vi "niLvFpga_StartFifo_sbRIO-9603.vi"(0 "session in":u32, 5 "channel":u32, 11 "error in":errorcluster) -> (4 "session out":u32, 15 "error out":errorcluster)   [LabVIEW 2020]
uses:
  <vilib>/rvi/interface/common/niFpgaWaitOnOcc.vi
  NiFpgaLv.dll
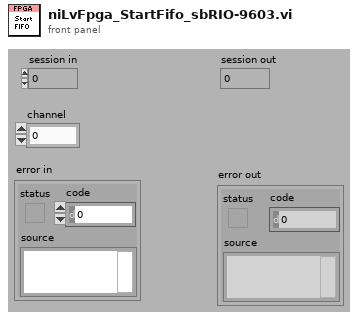
[diagram p1: front panel]
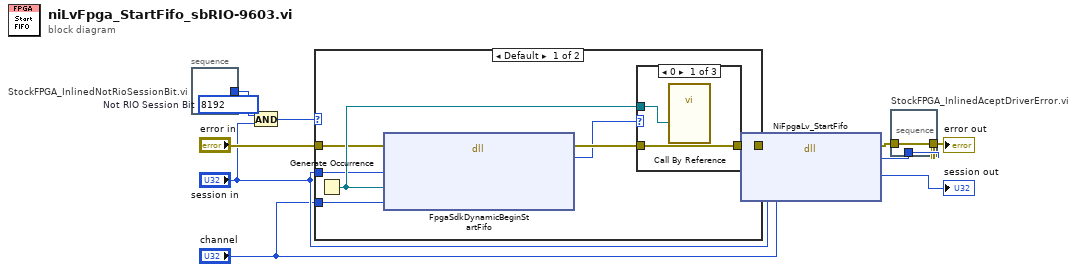
[diagram p0: block diagram]
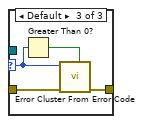
[diagram p4: hidden frame]
diagram:
  n1 = stacked-sequence "StockFPGA_InlinedNotRioSessionBit.vi" {
    tunnel: [w11] -> w3
    frame #0 {
      w11 = u32 8192  # Not RIO Session Bit
    }
  }
  n2 = And(x=w3, y="session in") -> (x .and. y?=w6:u32)
  n3 = case shown="Default" w6 {
    tunnel: "error in" -> [w15 w26]
    tunnel: [w14 w26] -> w4
    tunnel: "session in" -> [w13 _]
    tunnel: "channel" -> [w12 _]
    frame Default {
      n4 = Generate Occurrence() -> (w18:refnum<k4>)
      n5 = dll-call lib="LabVIEW" fn="FpgaSdkDynamicBeginStartFifo"(error in=w15, "session"=w13, "occurrence"=w18, "channel"=w12) -> (error out=w17:errorcluster, "status"=w16:i32)  [unwired: 5 in, 1 out]
      n6 = case shown="0" w16 {
        selector: w16 -> [_ _ w22]
        tunnel: [w20 w21 w24] -> w14
        tunnel: w17 -> [w20 w21 w25]
        tunnel: w18 -> [w19 _ _]
        frame 0 {
          n7 = call-by-ref "?"("occurrence"=w19) -> ()  [unwired: 16 in, 3 out]
        }
        frame -61167 {
          # "emulation case intentionally ignoring error"
        }
        frame Default {
          n8 = Greater Than 0?(x=w22) -> (x > 0?=w23:bool)
          n9 = call <vilib>:"Error Cluster From Error Code.vi"("is warning? (False)"=w23, "error in (no error)"=w25, "error code (0)"=w22) -> ("error out"=w24:errorcluster)  [unwired: 6 in]
        }
      }
    }
    frame 0 {
    }
  }
  n10 = dll-call lib="NiFpgaLv.*" fn="NiFpgaLv_StartFifo" label="niLvFpgaStartFifo"(error in=w4, "sessionID"="session in", "channel"="channel") -> (error out=w9:errorcluster, "status"=w7:i32, "sessionID"=→"session out":u32)  [unwired: 3 in, 1 out]
  n11 = stacked-sequence "StockFPGA_InlinedAceptDriverError.vi" {
    tunnel: w9 -> [w27]
    tunnel: w7 -> [w29]
    tunnel: [w28] -> w8
    frame #0 {
      n12 = case shown="Default" w29 {
        selector: w29 -> [_ w31]
        tunnel: [w30 w33] -> w28
        tunnel: w27 -> [w30 w34]
        frame 0 {
        }
        frame Default {
          n13 = Greater Than 0?(x=w31) -> (x > 0?=w32:bool)
          n14 = call <vilib>:"Error Cluster From Error Code.vi"("is warning? (False)"=w32, "error in (no error)"=w34, "error code (0)"=w31) -> ("error out"=w33:errorcluster)  [unwired: 6 in]
        }
      }
    }
  }
  "error out" <- w8
